vi "Test Test Fail if Expected API Call not Made.vi"(8 "error in (no error)":errorcluster, 11 "Test Case In":refnum<class "One Expectation Test.lvclass">) -> (0 "error out":errorcluster, 3 "Test Case Out":refnum<class "One Expectation Test.lvclass">)   [LabVIEW 2020, in "One Expectation Test.lvclass"]
uses:
  One Expectation Test.lvclass
  C:/Program Files (x86)/National Instruments/LabVIEW 2020/vi.lib/Astemes/LUnit/Test Case.lvclass
  Test Doubles/Test Interface Responsive Mock/Test Interface Mock.lvclass
  C:/git/astemes-lmock/source/Framework/Mock/Mock.lvclass
  source/Expectations/One/One Identical Inputs.vi
  One Expectation Test.lvclass/One Expectation Test.ctl
  source/Expectations/One/One.lvlib
  Expectation Test/Expectation Test.lvclass
  C:/git/astemes-lmock/tests/Test Doubles/Test Interface Responsive Mock/Test Interface Mock.lvclass
  C:/git/astemes-lmock/tests/Test Doubles/Test Interface/Test Interface.lvclass
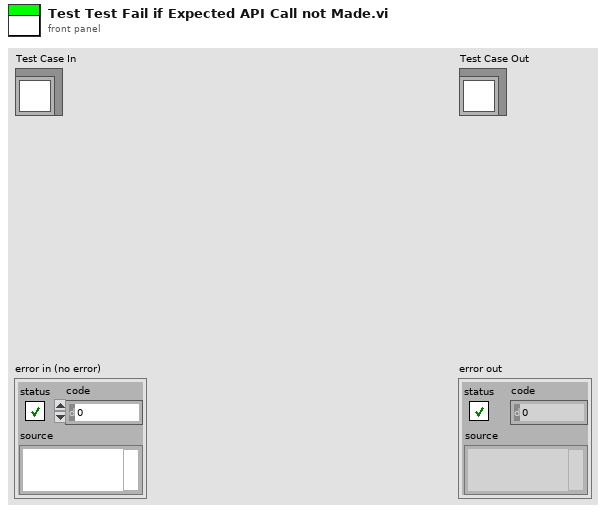
[diagram p1: front panel]
types:
  T1 = enum16{"", "Passed", "Failed", "Error", "Skipped", "Setup Error", "Broken", "Teardown Error"}
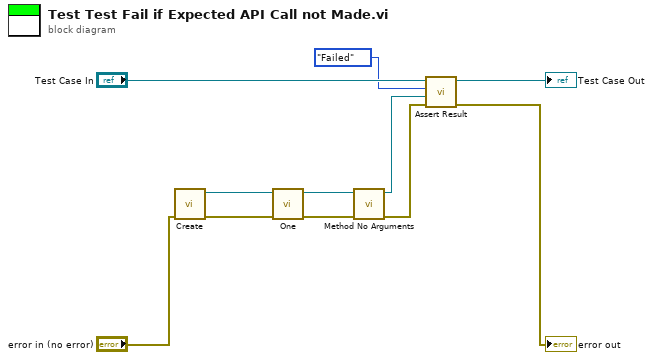
[diagram p0: block diagram]
diagram:
  n1 = call "Create.vi"("error in (no error)"="error in (no error)") -> ("error out"=w11:errorcluster, "Test Interface Mock Out"=w5:refnum<class "Test Interface Mock.lvclass">)  [unwired: 9 in]
  n2 = call-poly "One.vi"("error in (no error)"=w11, "Mock in"=w5) -> ("error out"=w10:errorcluster, "Mock out"=w4:refnum<class "Test Interface Mock.lvclass">)  [unwired: 8 in]
  n3 = call-dynamic "Method No Arguments.vi"("error in (no error)"=w10, "Mock In"=w4) -> ("error out"=w3:errorcluster, "Mock Out"=w2:refnum<class "Test Interface Mock.lvclass">)  [unwired: 8 in]
  n4 = call "Assert Result.vi"("error in (no error)"=w3, "Mock"=w2, "Status"=T1."Failed", "LUnit Test Case In"="Test Case In") -> ("error out"=→"error out":errorcluster, "LUnit Test Case Out"=→"Test Case Out":refnum<class "One Expectation Test.lvclass">)  [unwired: 6 in]
